vi "CTRE_CANifier_ConfigFactoryDefault.vi"(6 "timeoutMs":i32=50, 8 "error in":errorcluster, 11 "CANifierDevRef":T3) -> (0 "error out":errorcluster, 3 "CANifierDevRef":T3)   [LabVIEW 2019]
doc: "Configures all persistant settings to default"
uses:
  <vilib>/Rock Robotics/WPI/ThirdParty/Phoenix-LabVIEW/CANifier/CTRE_CANifier_DeviceRef.ctl
  <vilib>/Rock Robotics/WPI/ThirdParty/Phoenix-LabVIEW/CANifier/CTRE_CANifier_Configurables.ctl
  <vilib>/Rock Robotics/WPI/ThirdParty/Phoenix-LabVIEW/Controls/CTRE_Phoenix_CustomParamConfiguration.ctl
panel:
  in  "CANifier Configuration":T1={"velocityMeasurementPeriod"=100, "velocityMeasurementWindow"=64, "clearPositionOnLimitF"=FALSE, "clearPositionOnLimitR"=FALSE, "clearPositionOnLimitQuadIdx"=FALSE, "CustomParam"={"customParam0"=0, "customParam1"=0}} {"velocityMeasurementPeriod" items=["Period_1Ms"=1, "Period_2Ms"=2, "Period_5Ms"=5, "Period_10Ms"=10, "Period_20Ms"=20, "Period_25Ms"=25, "Period_50Ms"=50, "Period_100Ms"=100]}
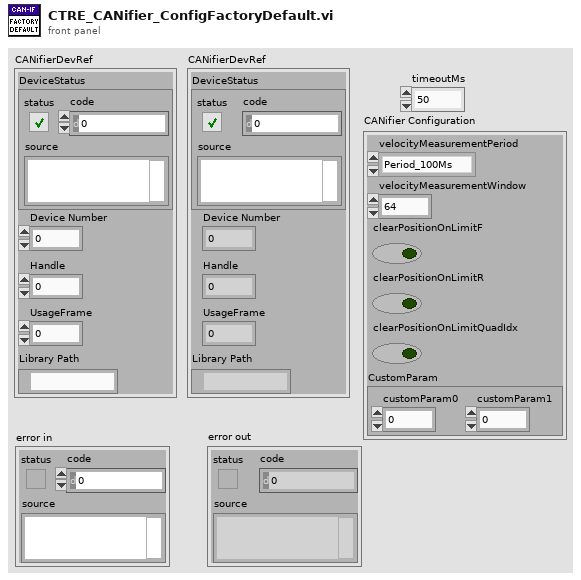
[diagram p1: front panel]
types:
  T1 = typedef "CTRE_CANifier_Configurables.ctl" = cluster{"velocityMeasurementPeriod":u16, "velocityMeasurementWindow":i32, "clearPositionOnLimitF":bool, "clearPositionOnLimitR":bool, "clearPositionOnLimitQuadIdx":bool, "CustomParam":T2}
  T2 = typedef "CTRE_Phoenix_CustomParamConfiguration.ctl" = cluster{"customParam0":i32, "customParam1":i32}
  T3 = typedef "CTRE_CANifier_DeviceRef.ctl" = cluster{"DeviceStatus":errorcluster, "Device Number":u8, "Handle":u64, "UsageFrame":u32, "Library Path":path}
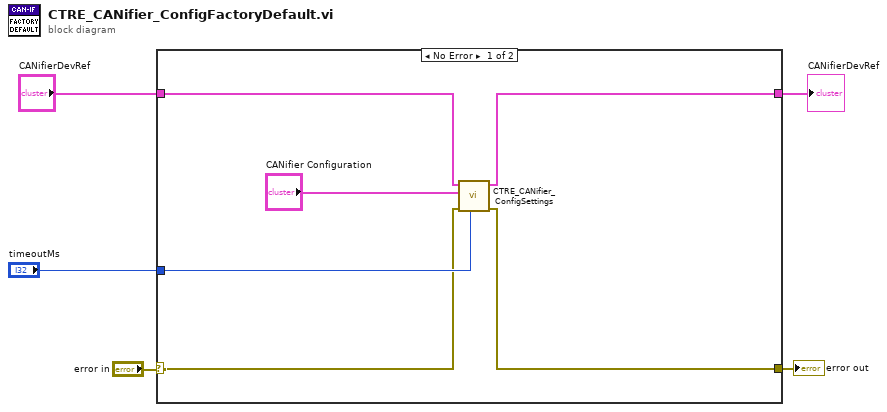
[diagram p0: block diagram]
diagram:
  n1 = case shown="No Error" "error in" {
    selector: "error in" -> [w8 w13]
    tunnel: [w7 w13] -> w4
    tunnel: "CANifierDevRef" -> [w11 w12]
    tunnel: [w10 w12] -> w2
    tunnel: "timeoutMs" -> [w9 _]
    frame No Error {
      n2 = call <vilib>:"CTRE_CANifier_ConfigSettings.vi"("timeoutMs"=w9, "error in (no error)"=w8, "CANifier Configuration"="CANifier Configuration", "CANifierDevRef"=w11) -> ("error out"=w7:errorcluster, "CANifierDevRef"=w10:T3)  [unwired: 6 in]
    }
    frame Error {
    }
  }
  "error out" <- w4
  "CANifierDevRef" <- w2
